vi "Autonomous Independent.vi"() -> ()   [LabVIEW 2017]
doc: "This VI is called when autonomous begins, and will automatically be terminated when autonomous ends. You can carry out timed or sensor driven robot movement independently without needing to return to the caller."
uses:
  <vilib>/Rock Robotics/WPI/Utilities/WPI_GetSetVariantRefNum.vi
  <vilib>/Rock Robotics/Network Tables/NT Read String.vi
  <vilib>/Rock Robotics/WPI/RobotDrive/WPI_RobotDriveArcadeDrive_Standard(NoSaturation).vi
  <vilib>/Rock Robotics/Network Tables/NT Write Numeric Array.vi
  Robot Global Data.vi
panel:
  out "Current Movement, for debugging":T1 {"Y Joystick Value" scale=1.0..-1.0; "X Joystick Value" scale=-1.0..1.0}
  in  "Array of robot movements":T2(array[cluster])=[{"X Joystick Value"=0.39393939393939403, "Y Joystick Value"=0.0, "Delay (sec)"=1.0, "Movement Name"="turn"}, {"X Joystick Value"=-0.3737373737373737, "Y Joystick Value"=0.0, "Delay (sec)"=1.0, "Movement Name"="turn back"}] {"Y Joystick Value" scale=1.0..-1.0; "X Joystick Value" scale=-1.0..1.0}
  # "Be sure to right-click and choose Data Operations>>Make Current Value default if you want to save the array values with the VI"
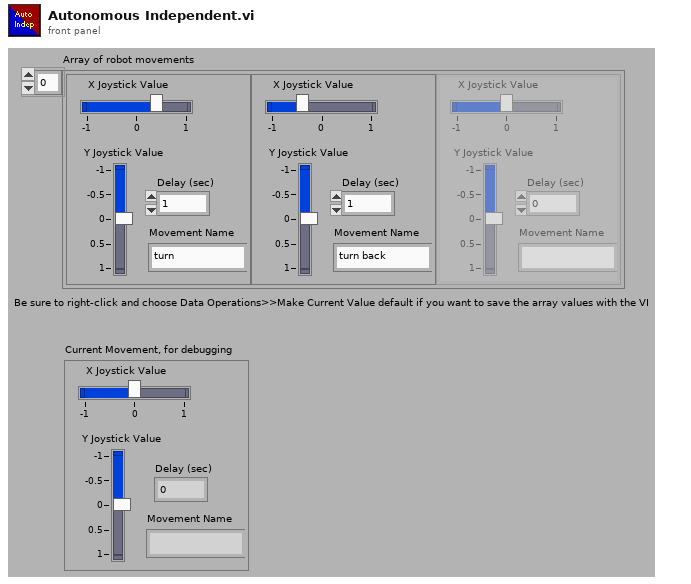
[diagram p1: front panel]
types:
  T1 = cluster{"X Joystick Value":dbl, "Y Joystick Value":dbl, "Delay (sec)":dbl, "Movement Name":string}
  T2 = cluster{"X Joystick Value":dbl, "Y Joystick Value":dbl, "Delay (sec)":dbl, "Movement Name":string}[]
  T3 = typedef "WPI_JoystickDevRef.ctl" = cluster{"Device":T4}
  T4 = typedef "WPI_JoystickDeviceEnum.ctl" = enum16{"USB 0", "USB 1", "USB 2", "USB 3", "USB 4", "USB 5"}
  T5 = typedef "WPI_RobotDriveDevRef.ctl" = cluster{"DevStatus":errorcluster, "Motors[]":T6[], "Square Inputs":bool, "Max Output":dbl}
  T6 = typedef "WPI_MotorControlDeviceRef.ctl" = cluster{"DeviceStatus":errorcluster, "Type":T7, "PWM":cluster{"PWM Channel":T8, "DeadBand":T9}, "CAN":cluster{"Device Number":u8, "SetOutput VI Ref":variant, "GetOutput VI Ref":variant, "Enable VI Ref":variant, "Disable VI Ref":variant, "Data":variant}, "Invert":bool, "DIO PWM":cluster{"PWM \"Enable\" Channel":T8, "DIOChannel":T10, "PWM Rate":dbl}}
  T7 = typedef "WPI_MotorControlType.ctl" = enum16{"PWM", "CAN", "DIO PWM"}
  T8 = typedef "FPGA_DIOPWMChannel.ctl" = enum8{"PWM 0", "PWM 1", "PWM 2", "PWM 3", "PWM 4", "PWM 5", "PWM 6", "PWM 7", "PWM 8", "PWM 9", "PWM MXP 0", "PWM MXP 1", "PWM MXP 2", "PWM MXP 3", "PWM MXP 4", "PWM MXP 5", "PWM MXP 6", "PWM MXP 7", "PWM MXP 8", "PWM MXP 9", "Invalid"}
  T9 = typedef "WPI_PWMDeadband.ctl" = cluster{"Name":string, "maxPositivePwm":i32, "minPositivePwm":i32, "centerPwm":i32, "maxNegativePwm":i32, "minNegativePwm":i32, "angularRange":u16}
  T10 = typedef "FPGA_DIOChannel.ctl" = enum8{"DIO 0", "DIO 1", "DIO 2", "DIO 3", "DIO 4", "DIO 5", "DIO 6", "DIO 7", "DIO 8", "DIO 9", "DIO MXP 0", "DIO MXP 1", "DIO MXP 2", "DIO MXP 3", "DIO MXP 4", "DIO MXP 5", "DIO MXP 6", "DIO MXP 7", "DIO MXP 8", "DIO MXP 9", "DIO MXP 10", "DIO MXP 11", "DIO MXP 12", "DIO MXP 13", "DIO MXP 14", "DIO MXP 15", "SPI Port CS1", "SPI Port CS2", "SPI Port CS3", "SPI Port MISO", "SPI Port MOSI", "Invalid"}
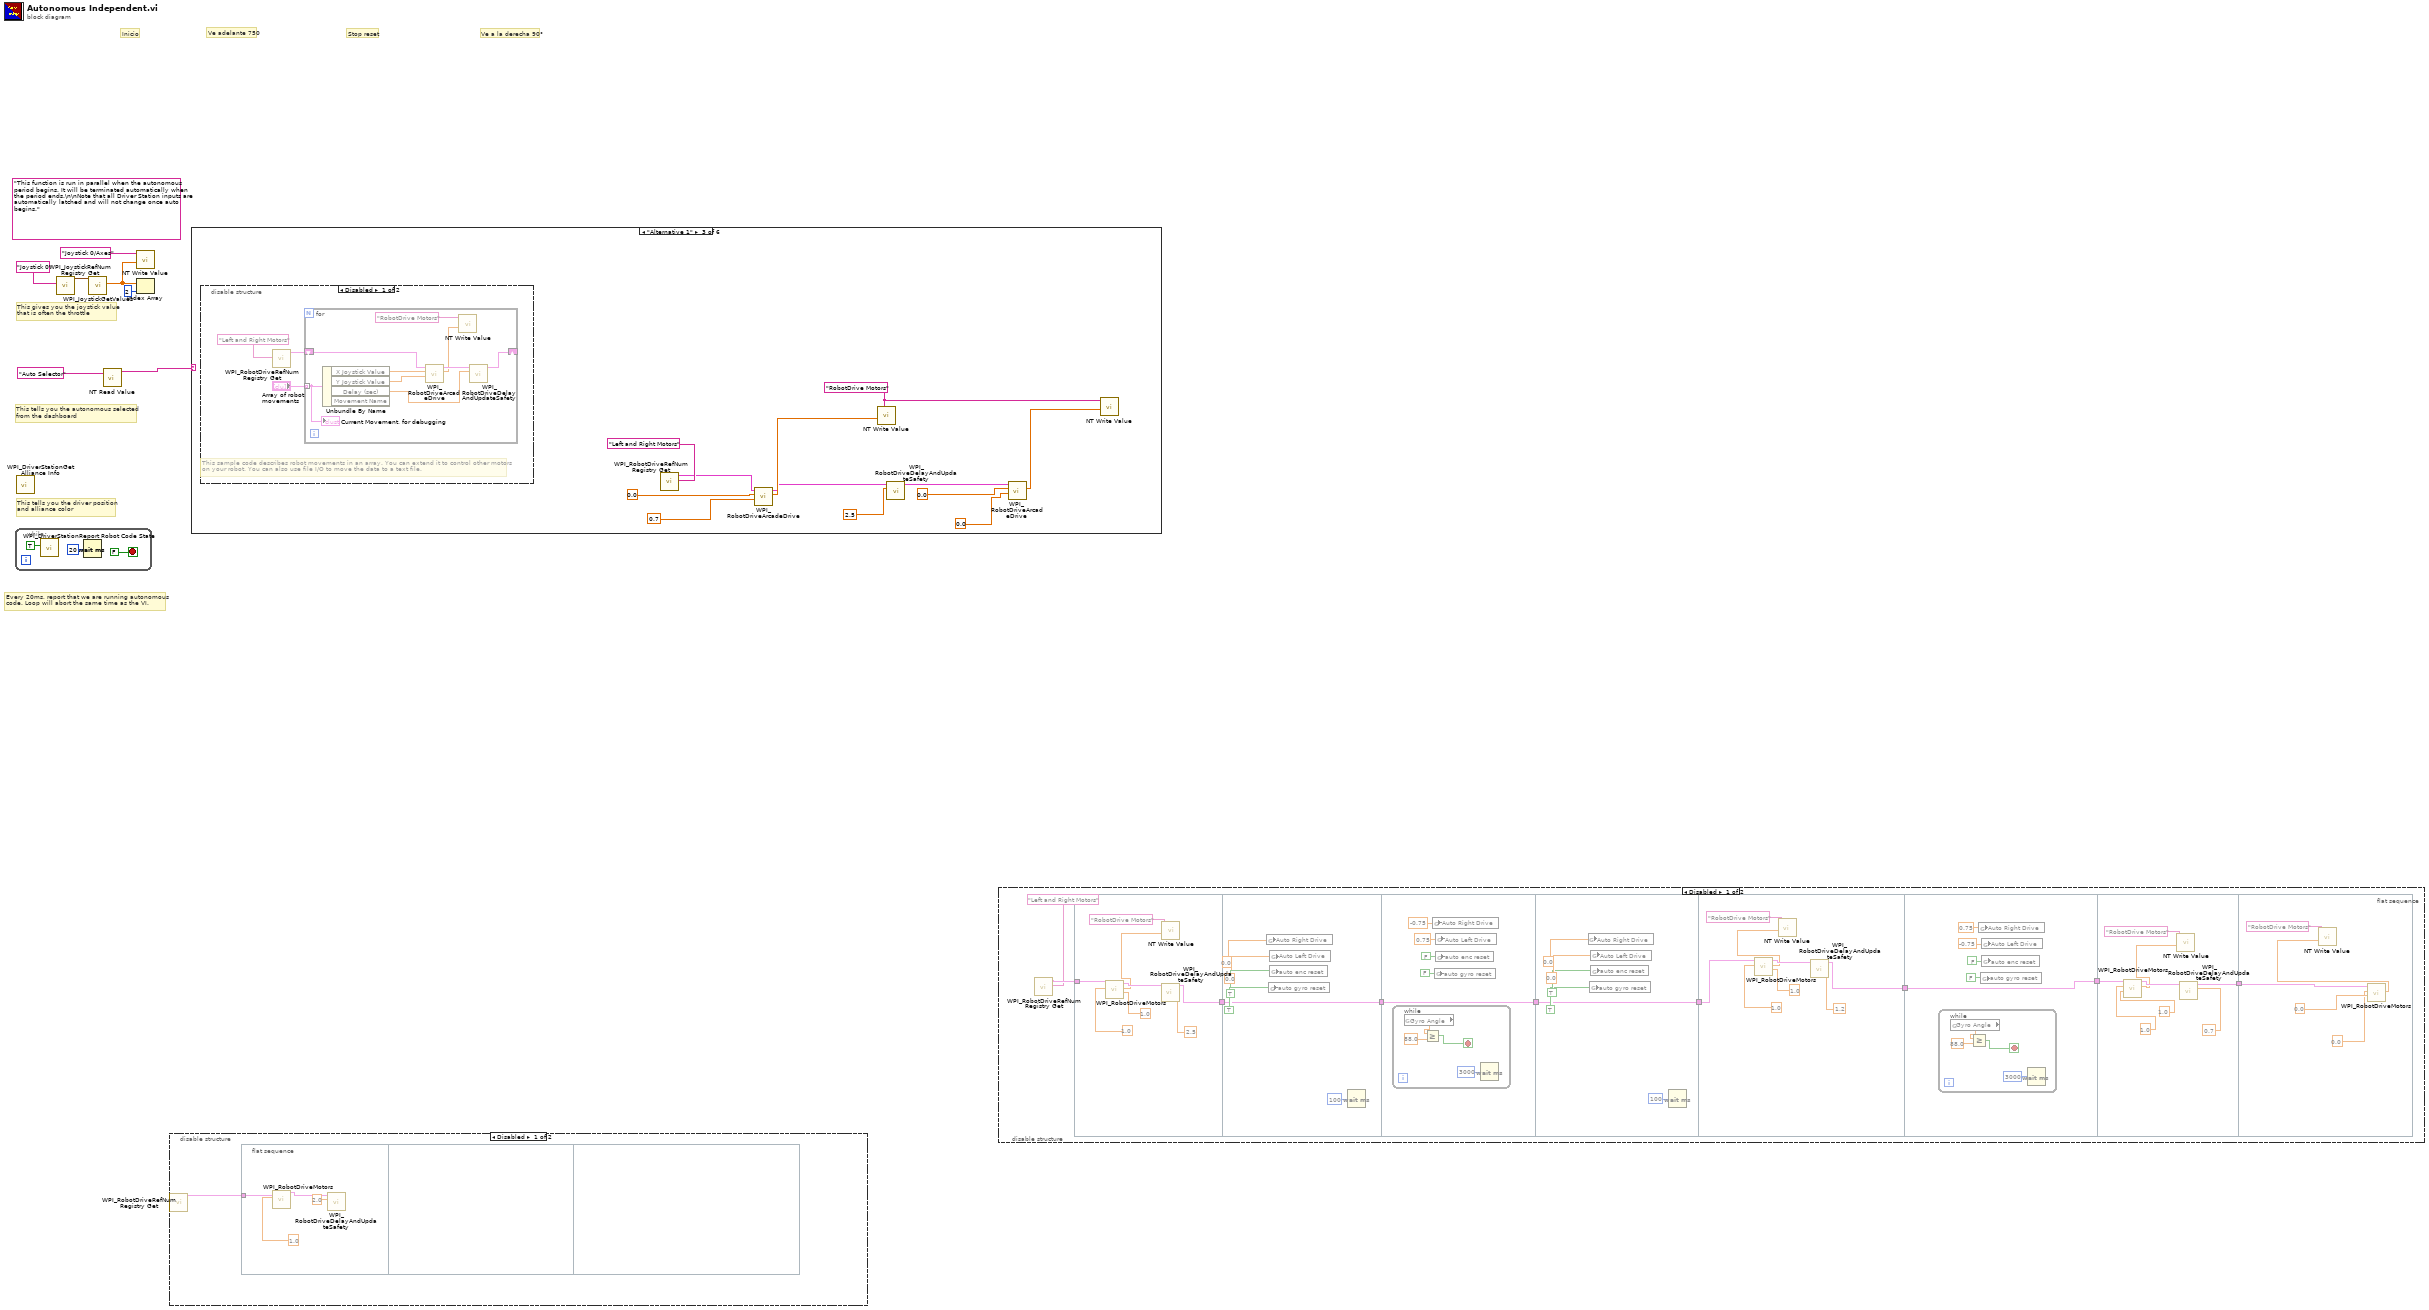
[diagram p0: block diagram]
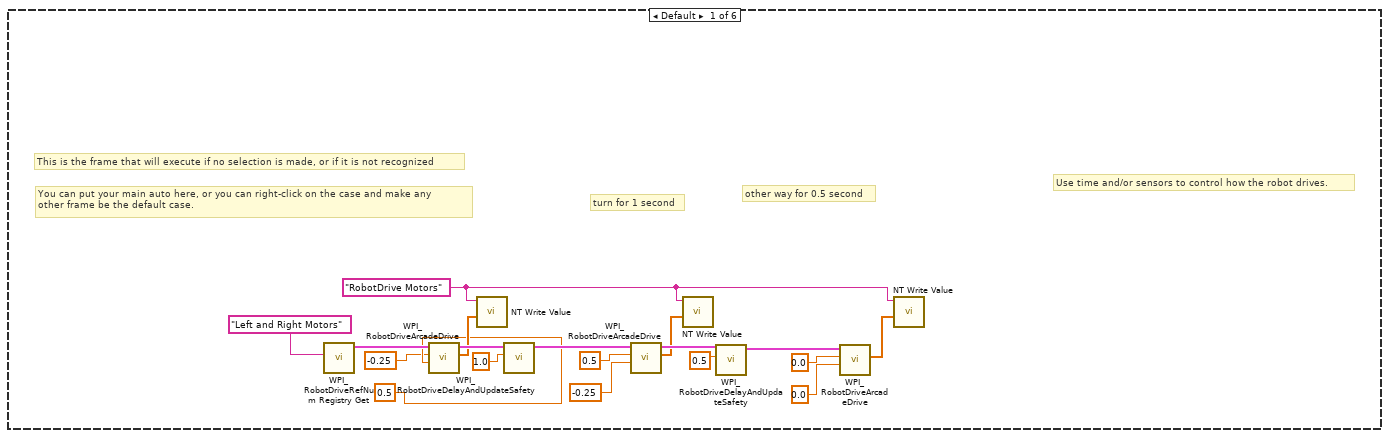
[diagram p4: hidden frame]
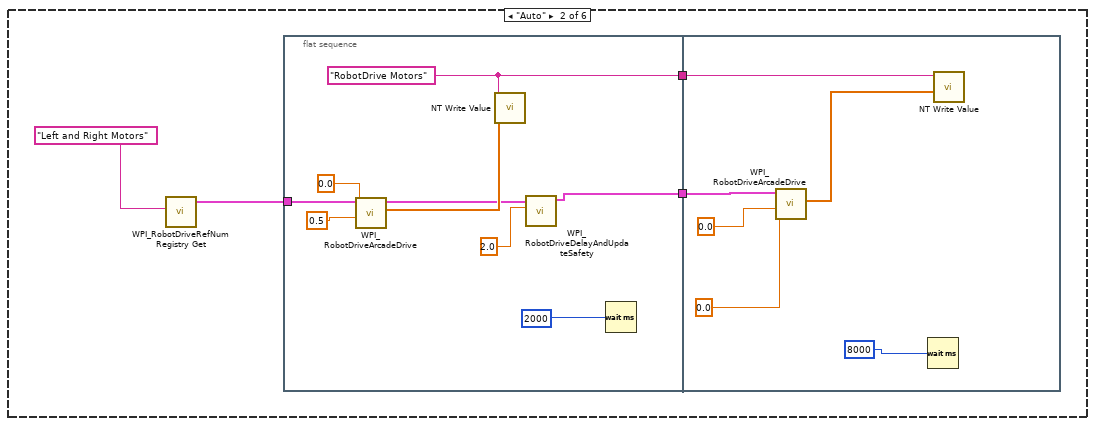
[diagram p5: hidden frame]
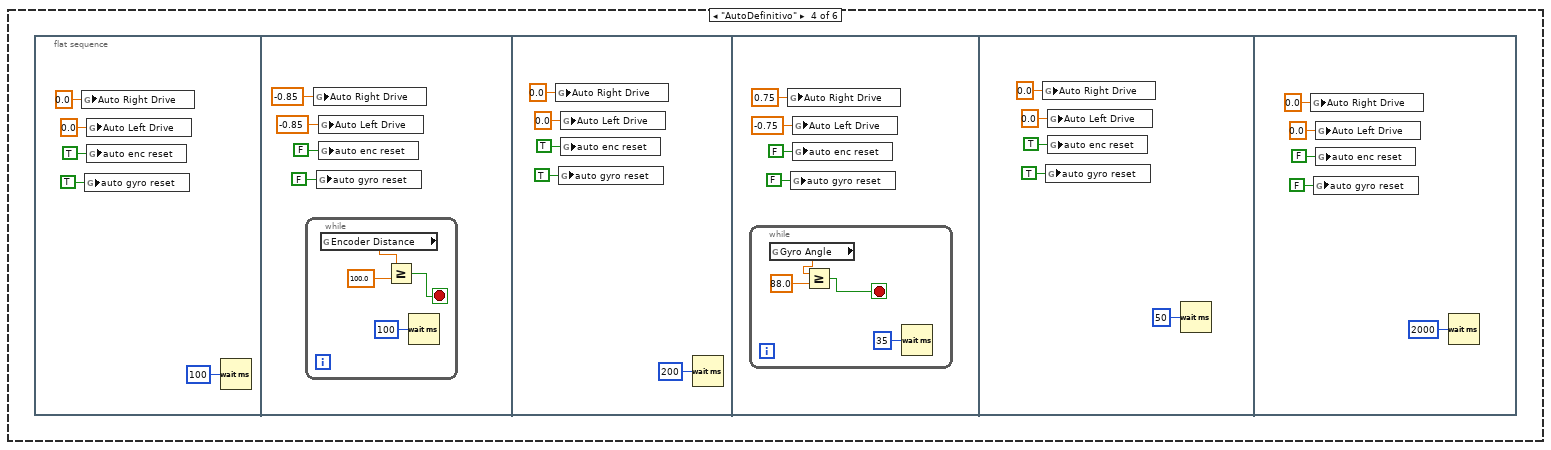
[diagram p7: hidden frame]
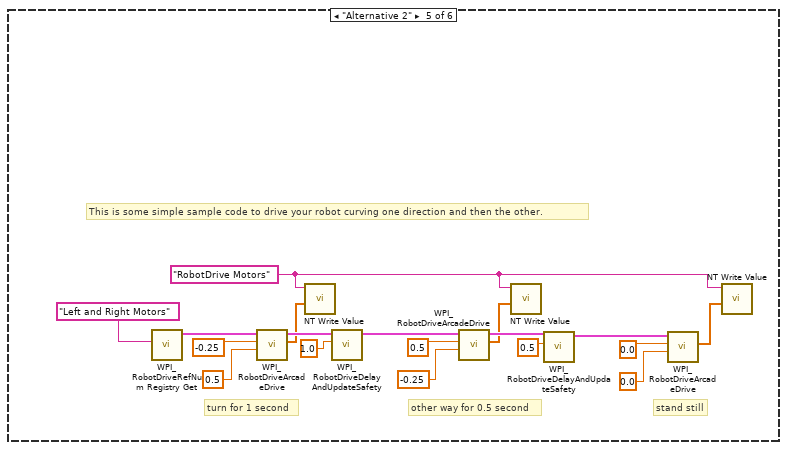
[diagram p8: hidden frame]
diagram:
  (unwired) "This function is run in parallel when the autonomous period begins. It will be terminated automatically when the period ends.\n\nNote that all Driver Station inputs are automatically latched and will not change once auto begins."
  # "Ve a la derecha 90°"
  # "Stop reset"
  # "Ve adelante 750"
  # "Inicio"
  # "This tells you the autonomous selected\nfrom the dashboard"
  # "Every 20ms, report that we are running autonomous\ncode. Loop will abort the same time as the VI."
  # "This gives you the joystick value\nthat is often the throttle"
  # "This tells you the driver position\nand alliance color"
  n1 = while {
    stop <- FALSE stop-if-true
    n2 = call <vilib>:"WPI_DriverStationReport Robot Code State.vi"("Autonomous"=TRUE) -> ()  [unwired: 10 in, 1 out]
    n3 = Wait (ms)(milliseconds to wait=u32 20) -> ()  [unwired: 1 out]
  }
  n4 = call <vilib>:"WPI_DriverStationGet Alliance Info.vi"() -> ()  [unwired: 12 out]
  n5 = call <vilib>:"WPI_JoystickRefNum Registry Get.vi"("refnum name"="Joystick 0") -> ("JoystickDevRef"=w6:T3)  [unwired: 1 in, 9 out]
  n6 = call <vilib>:"WPI_JoystickGetValues.vi"("JoystickDevRef"=w6) -> ("Axes"=w2:dbl[])  [unwired: 6 in, 4 out]
  n7 = call-poly <vilib>:"NT Read Value.vi"("Name"="Auto Selector") -> ("String"=w3:string)  [unwired: 9 in, 1 out]
  n8 = call-poly <vilib>:"NT Write Value.vi"("Numeric Array"=w2, "Name"="Joystick 0/Axes") -> ()  [unwired: 9 in, 1 out]
  n9 = Index Array(array=w2, index=2) -> ()  [unwired: 1 out]
  n10 = disable-structure shown="Disabled" {
    frame Disabled {
      n11 = call <vilib>:"WPI_RobotDriveRefNum Registry Get.vi"() -> ("RobotDriveDevRef"=w11:T5)  [unwired: 10 in, 1 out]
      n12 = flat-sequence {
        tunnel: w11 -> [w15]
        frame #0 {
          n13 = call <vilib>:"WPI_RobotDriveMotors.vi"("LeftSpeed"=1.0, "RobotDriveDevRef"=w15) -> ("RobotDriveDevRef"=w14:T5)  [unwired: 7 in, 2 out]
          n14 = call <vilib>:"WPI_RobotDriveDelayAndUpdateSafety.vi"("Delay (s)"=2.0, "RobotDriveDevRef"=w14) -> ()  [unwired: 8 in, 2 out]
        }
        frame #1 {
        }
        frame #2 {
        }
      }
    }
    frame Enabled {
    }
  }
  n15 = case shown="\"Alternative 1\"" w3 {
    frame Default {
      w25 = "RobotDrive Motors" ("Name")
      # "other way for 0.5 second"
      # "turn for 1 second"
      # "Use time and/or sensors to control how the robot drives."
      # "You can put your main auto here, or you can right-click on the case and make any\nother frame be the default case."
      # "This is the frame that will execute if no selection is made, or if it is not recognized"
      n16 = call <vilib>:"WPI_RobotDriveRefNum Registry Get.vi"("refnum name"="Left and Right Motors") -> ("RobotDriveDevRef"=w33:T5)  [unwired: 1 in, 9 out]
      n17 = call-poly <vilib>:"WPI_RobotDriveArcadeDrive.vi"("Y axis value"=0.5 ("X axis value"), "X axis value"=-0.25, "RobotDriveDevRef"=w33) -> ("Motor Values"=w26:dbl[], "RobotDriveDevRef"=w29:T5)  [unwired: 1 in, 6 out]
      n18 = call-poly <vilib>:"NT Write Value.vi"("Numeric Array"=w26, "Name"=w25) -> ()  [unwired: 9 in, 1 out]
      n19 = call <vilib>:"WPI_RobotDriveDelayAndUpdateSafety.vi"("Delay (s)"=1.0, "RobotDriveDevRef"=w29) -> ("RobotDriveDevRef 2"=w30:T5)  [unwired: 8 in, 1 out]
      n20 = call-poly <vilib>:"WPI_RobotDriveArcadeDrive.vi"("Y axis value"=-0.25 ("X axis value"), "X axis value"=0.5, "RobotDriveDevRef"=w30) -> ("Motor Values"=w27:dbl[], "RobotDriveDevRef"=w31:T5)  [unwired: 1 in, 6 out]
      n21 = call-poly <vilib>:"NT Write Value.vi"("Numeric Array"=w27, "Name"=w25) -> ()  [unwired: 9 in, 1 out]
      n22 = call <vilib>:"WPI_RobotDriveDelayAndUpdateSafety.vi"("Delay (s)"=0.5, "RobotDriveDevRef"=w31) -> ("RobotDriveDevRef 2"=w32:T5)  [unwired: 8 in, 1 out]
      n23 = call-poly <vilib>:"WPI_RobotDriveArcadeDrive.vi"("Y axis value"=0.0 ("X axis value"), "X axis value"=0.0, "RobotDriveDevRef"=w32) -> ("Motor Values"=w28:dbl[])  [unwired: 1 in, 7 out]
      n24 = call-poly <vilib>:"NT Write Value.vi"("Numeric Array"=w28, "Name"=w25) -> ()  [unwired: 9 in, 1 out]
    }
    frame "Auto" {
      n25 = call <vilib>:"WPI_RobotDriveRefNum Registry Get.vi"("refnum name"="Left and Right Motors") -> ("RobotDriveDevRef"=w36:T5)  [unwired: 9 in, 1 out]
      n26 = flat-sequence {
        tunnel: w36 -> [w46]
        tunnel: [w39] -> w35
        tunnel: [w44] -> w34
        tunnel: w35 -> [w52]
        tunnel: w34 -> [w50]
        frame #0 {
          w44 = "RobotDrive Motors" ("Name")
          n27 = call-poly <vilib>:"WPI_RobotDriveArcadeDrive.vi"("Y axis value"=0.5 ("X axis value"), "X axis value"=0.0, "RobotDriveDevRef"=w46) -> ("Motor Values"=w45:dbl[], "RobotDriveDevRef"=w41:T5)  [unwired: 6 in, 1 out]
          n28 = call-poly <vilib>:"NT Write Value.vi"("Numeric Array"=w45, "Name"=w44) -> ()  [unwired: 9 in, 1 out]
          n29 = call <vilib>:"WPI_RobotDriveDelayAndUpdateSafety.vi"("Delay (s)"=2.0, "RobotDriveDevRef"=w41) -> ("RobotDriveDevRef 2"=w39:T5)  [unwired: 8 in, 1 out]
          n30 = Wait (ms)(milliseconds to wait=2000) -> ()  [unwired: 1 out]
        }
        frame #1 {
          n31 = call-poly <vilib>:"WPI_RobotDriveArcadeDrive.vi"("Y axis value"=0.0, "X axis value"=0.0, "RobotDriveDevRef"=w52) -> ("Motor Values"=w49:dbl[])  [unwired: 6 in, 2 out]
          n32 = Wait (ms)(milliseconds to wait=8000) -> ()  [unwired: 1 out]
          n33 = call-poly <vilib>:"NT Write Value.vi"("Numeric Array"=w49, "Name"=w50) -> ()  [unwired: 9 in, 1 out]
        }
      }
    }
    frame "Alternative 1" {
      w56 = "RobotDrive Motors" ("Name")
      n34 = disable-structure shown="Disabled" {
        frame Disabled {
          # "This sample code describes robot movements in an array. You can extend it to control other motors\non your robot. You can also use file I/O to move the data to a text file."
          n35 = call <vilib>:"WPI_RobotDriveRefNum Registry Get.vi"("refnum name"="Left and Right Motors") -> ("RobotDriveDevRef"=w66:T5)  [unwired: 1 in, 9 out]
          n36 = for {
            shift-right: [w74] -> _
            shift-left: w66 -> [w75]
            tunnel: "Array of robot movements" -> [w70] mode=indexing
            n37 = Unbundle By Name(w70) -> ("X Joystick Value"=w73:dbl, "Y Joystick Value"=w72:dbl, "Delay (sec)"=w71:dbl)  [unwired: 1 out]
            n38 = call-poly <vilib>:"WPI_RobotDriveArcadeDrive.vi"("Y axis value"=w72, "X axis value"=w73, "RobotDriveDevRef"=w75) -> ("Motor Values"=w68:dbl[], "RobotDriveDevRef"=w76:T5)  [unwired: 1 in, 6 out]
            n39 = call-poly <vilib>:"NT Write Value.vi"("Numeric Array"=w68, "Name"="RobotDrive Motors") -> ()  [unwired: 9 in, 1 out]
            n40 = call <vilib>:"WPI_RobotDriveDelayAndUpdateSafety.vi"("Delay (s)"=w71, "RobotDriveDevRef"=w76) -> ("RobotDriveDevRef 2"=w74:T5)  [unwired: 8 in, 1 out]
            "Current Movement, for debugging" <- w70
          }
        }
        frame Enabled {
        }
      }
      n41 = call <vilib>:"WPI_RobotDriveRefNum Registry Get.vi"("refnum name"="Left and Right Motors") -> ("RobotDriveDevRef"=w61:T5)  [unwired: 9 in, 1 out]
      n42 = call-poly <vilib>:"WPI_RobotDriveArcadeDrive.vi"("Y axis value"=0.7 ("RightSpeed"), "X axis value"=0.0 ("LeftSpeed"), "RobotDriveDevRef"=w61) -> ("Motor Values"=w59:dbl[], "RobotDriveDevRef"=w58:T5)  [unwired: 6 in, 1 out]
      n43 = call-poly <vilib>:"NT Write Value.vi"("Numeric Array"=w59, "Name"=w56) -> ()  [unwired: 9 in, 1 out]
      n44 = call <vilib>:"WPI_RobotDriveDelayAndUpdateSafety.vi"("Delay (s)"=2.5, "RobotDriveDevRef"=w58) -> ("RobotDriveDevRef 2"=w57:T5)  [unwired: 8 in, 1 out]
      n45 = call-poly <vilib>:"WPI_RobotDriveArcadeDrive.vi"("Y axis value"=0.0 ("LeftSpeed"), "X axis value"=0.0 ("RightSpeed"), "RobotDriveDevRef"=w57) -> ("Motor Values"=w53:dbl[])  [unwired: 6 in, 2 out]
      n46 = call-poly <vilib>:"NT Write Value.vi"("Numeric Array"=w53, "Name"=w56) -> ()  [unwired: 9 in, 1 out]
    }
    frame "AutoDefinitivo" {
      n47 = flat-sequence {
        frame #0 {
          n48 = global write "Robot Global Data.vi" "Auto Right Drive"(0.0 ("Auto Right Drive")) -> ()
          n49 = global write "Robot Global Data.vi" "auto gyro reset"(TRUE ("auto gyro reset")) -> ()
          n50 = global write "Robot Global Data.vi" "Auto Left Drive"(0.0 ("Auto Left Drive")) -> ()
          n51 = global write "Robot Global Data.vi" "auto enc reset"(TRUE ("auto enc reset")) -> ()
          n52 = Wait (ms)(milliseconds to wait=u32 100) -> ()  [unwired: 1 out]
        }
        frame #1 {
          n53 = while {
            stop <- w87 stop-if-true
            n54 = global read "Robot Global Data.vi" "Encoder Distance"() -> (w89:dbl)
            n55 = Greater Or Equal?(x=w89, y=100.0) -> (x >= y?=w87:bool)
            n56 = Wait (ms)(milliseconds to wait=u32 100) -> ()  [unwired: 1 out]
          }
          n57 = global write "Robot Global Data.vi" "Auto Right Drive"(-0.85 ("Auto Right Drive")) -> ()
          n58 = global write "Robot Global Data.vi" "auto gyro reset"(FALSE ("auto gyro reset")) -> ()
          n59 = global write "Robot Global Data.vi" "Auto Left Drive"(-0.85 ("Auto Left Drive")) -> ()
          n60 = global write "Robot Global Data.vi" "auto enc reset"(FALSE ("auto enc reset")) -> ()
        }
        frame #2 {
          n61 = global write "Robot Global Data.vi" "Auto Right Drive"(0.0 ("Auto Right Drive")) -> ()
          n62 = global write "Robot Global Data.vi" "auto gyro reset"(TRUE ("auto gyro reset")) -> ()
          n63 = global write "Robot Global Data.vi" "Auto Left Drive"(0.0 ("Auto Left Drive")) -> ()
          n64 = global write "Robot Global Data.vi" "auto enc reset"(TRUE ("auto enc reset")) -> ()
          n65 = Wait (ms)(milliseconds to wait=u32 200) -> ()  [unwired: 1 out]
        }
        frame #3 {
          n66 = while {
            stop <- w100 stop-if-true
            n67 = global read "Robot Global Data.vi" "Gyro Angle"() -> (w102:dbl)
            n68 = Greater Or Equal?(x=w102, y=88.0) -> (x >= y?=w100:bool)
            n69 = Wait (ms)(milliseconds to wait=u32 35) -> ()  [unwired: 1 out]
          }
          n70 = global write "Robot Global Data.vi" "Auto Right Drive"(0.75 ("Auto Right Drive")) -> ()
          n71 = global write "Robot Global Data.vi" "auto gyro reset"(FALSE ("auto gyro reset")) -> ()
          n72 = global write "Robot Global Data.vi" "Auto Left Drive"(-0.75 ("Auto Left Drive")) -> ()
          n73 = global write "Robot Global Data.vi" "auto enc reset"(FALSE ("auto enc reset")) -> ()
        }
        frame #4 {
          n74 = global write "Robot Global Data.vi" "Auto Right Drive"(0.0 ("Auto Right Drive")) -> ()
          n75 = global write "Robot Global Data.vi" "auto gyro reset"(TRUE ("auto gyro reset")) -> ()
          n76 = global write "Robot Global Data.vi" "Auto Left Drive"(0.0 ("Auto Left Drive")) -> ()
          n77 = global write "Robot Global Data.vi" "auto enc reset"(TRUE ("auto enc reset")) -> ()
          n78 = Wait (ms)(milliseconds to wait=u32 50) -> ()  [unwired: 1 out]
        }
        frame #5 {
          n79 = global write "Robot Global Data.vi" "Auto Right Drive"(0.0 ("Auto Right Drive")) -> ()
          n80 = global write "Robot Global Data.vi" "auto gyro reset"(FALSE ("auto gyro reset")) -> ()
          n81 = global write "Robot Global Data.vi" "Auto Left Drive"(0.0 ("Auto Left Drive")) -> ()
          n82 = global write "Robot Global Data.vi" "auto enc reset"(FALSE ("auto enc reset")) -> ()
          n83 = Wait (ms)(milliseconds to wait=u32 2000) -> ()  [unwired: 1 out]
        }
      }
    }
    frame "Alternative 2" {
      w114 = "RobotDrive Motors" ("Name")
      # "This is some simple sample code to drive your robot curving one direction and then the other."
      # "stand still"
      # "other way for 0.5 second"
      # "turn for 1 second"
      n84 = call <vilib>:"WPI_RobotDriveRefNum Registry Get.vi"("refnum name"="Left and Right Motors") -> ("RobotDriveDevRef"=w130:T5)  [unwired: 1 in, 9 out]
      n85 = call-poly <vilib>:"WPI_RobotDriveArcadeDrive.vi"("Y axis value"=0.5 ("X axis value"), "X axis value"=-0.25, "RobotDriveDevRef"=w130) -> ("Motor Values"=w113:dbl[], "RobotDriveDevRef"=w123:T5)  [unwired: 1 in, 6 out]
      n86 = call-poly <vilib>:"NT Write Value.vi"("Numeric Array"=w113, "Name"=w114) -> ()  [unwired: 9 in, 1 out]
      n87 = call <vilib>:"WPI_RobotDriveDelayAndUpdateSafety.vi"("Delay (s)"=1.0, "RobotDriveDevRef"=w123) -> ("RobotDriveDevRef 2"=w124:T5)  [unwired: 8 in, 1 out]
      n88 = call-poly <vilib>:"WPI_RobotDriveArcadeDrive.vi"("Y axis value"=-0.25 ("X axis value"), "X axis value"=0.5, "RobotDriveDevRef"=w124) -> ("Motor Values"=w115:dbl[], "RobotDriveDevRef"=w125:T5)  [unwired: 1 in, 6 out]
      n89 = call-poly <vilib>:"NT Write Value.vi"("Numeric Array"=w115, "Name"=w114) -> ()  [unwired: 9 in, 1 out]
      n90 = call <vilib>:"WPI_RobotDriveDelayAndUpdateSafety.vi"("Delay (s)"=0.5, "RobotDriveDevRef"=w125) -> ("RobotDriveDevRef 2"=w126:T5)  [unwired: 8 in, 1 out]
      n91 = call-poly <vilib>:"WPI_RobotDriveArcadeDrive.vi"("Y axis value"=0.0 ("X axis value"), "X axis value"=0.0, "RobotDriveDevRef"=w126) -> ("Motor Values"=w116:dbl[])  [unwired: 1 in, 7 out]
      n92 = call-poly <vilib>:"NT Write Value.vi"("Numeric Array"=w116, "Name"=w114) -> ()  [unwired: 9 in, 1 out]
    }
    frame "Your Turn" {
    }
  }
  n93 = disable-structure shown="Disabled" {
    frame Disabled {
      n94 = call <vilib>:"WPI_RobotDriveRefNum Registry Get.vi"("refnum name"="Left and Right Motors") -> ("RobotDriveDevRef"=w132:T5)  [unwired: 9 in, 1 out]
      n95 = flat-sequence {
        tunnel: w132 -> [w144]
        tunnel: [w142] -> w139
        tunnel: w139 -> [w148]
        tunnel: [w148] -> w138
        tunnel: [w154] -> w137
        tunnel: w138 -> [w154]
        tunnel: [w163] -> w136
        tunnel: w137 -> [w163]
        tunnel: w136 -> [w172]
        tunnel: [w171] -> w135
        tunnel: [w177] -> w134
        tunnel: w135 -> [w177]
        tunnel: w134 -> [w189]
        tunnel: [w188] -> w133
        tunnel: w133 -> [w196]
        frame #0 {
          n96 = call <vilib>:"WPI_RobotDriveMotors.vi"("RightSpeed"=1.0, "LeftSpeed"=1.0, "RobotDriveDevRef"=w144) -> ("Motor Values"=w141:dbl[], "RobotDriveDevRef"=w147:T5)  [unwired: 6 in, 1 out]
          n97 = call <vilib>:"WPI_RobotDriveDelayAndUpdateSafety.vi"("Delay (s)"=2.5, "RobotDriveDevRef"=w147) -> ("RobotDriveDevRef 2"=w142:T5)  [unwired: 8 in, 1 out]
          n98 = call-poly <vilib>:"NT Write Value.vi"("Numeric Array"=w141, "Name"="RobotDrive Motors") -> ()  [unwired: 9 in, 1 out]
        }
        frame #1 {
          n99 = global write "Robot Global Data.vi" "Auto Right Drive"(0.0 ("Auto Right Drive")) -> ()
          n100 = global write "Robot Global Data.vi" "auto gyro reset"(TRUE ("auto gyro reset")) -> ()
          n101 = global write "Robot Global Data.vi" "Auto Left Drive"(0.0 ("Auto Left Drive")) -> ()
          n102 = global write "Robot Global Data.vi" "auto enc reset"(TRUE ("auto enc reset")) -> ()
          n103 = Wait (ms)(milliseconds to wait=u32 100) -> ()  [unwired: 1 out]
        }
        frame #2 {
          n104 = while {
            stop <- w160 stop-if-true
            n105 = global read "Robot Global Data.vi" "Gyro Angle"() -> (w162:dbl)
            n106 = Greater Or Equal?(x=w162, y=88.0) -> (x >= y?=w160:bool)
            n107 = Wait (ms)(milliseconds to wait=u32 3000) -> ()  [unwired: 1 out]
          }
          n108 = global write "Robot Global Data.vi" "Auto Right Drive"(-0.75 ("Auto Right Drive")) -> ()
          n109 = global write "Robot Global Data.vi" "auto gyro reset"(FALSE ("auto gyro reset")) -> ()
          n110 = global write "Robot Global Data.vi" "Auto Left Drive"(0.75 ("Auto Left Drive")) -> ()
          n111 = global write "Robot Global Data.vi" "auto enc reset"(FALSE ("auto enc reset")) -> ()
        }
        frame #3 {
          n112 = global write "Robot Global Data.vi" "Auto Right Drive"(0.0 ("Auto Right Drive")) -> ()
          n113 = global write "Robot Global Data.vi" "auto gyro reset"(TRUE ("auto gyro reset")) -> ()
          n114 = global write "Robot Global Data.vi" "Auto Left Drive"(0.0 ("Auto Left Drive")) -> ()
          n115 = global write "Robot Global Data.vi" "auto enc reset"(TRUE ("auto enc reset")) -> ()
          n116 = Wait (ms)(milliseconds to wait=u32 100) -> ()  [unwired: 1 out]
        }
        frame #4 {
          n117 = call <vilib>:"WPI_RobotDriveMotors.vi"("RightSpeed"=1.0, "LeftSpeed"=1.0, "RobotDriveDevRef"=w172) -> ("Motor Values"=w169:dbl[], "RobotDriveDevRef"=w173:T5)  [unwired: 6 in, 1 out]
          n118 = call-poly <vilib>:"NT Write Value.vi"("Numeric Array"=w169, "Name"="RobotDrive Motors") -> ()  [unwired: 9 in, 1 out]
          n119 = call <vilib>:"WPI_RobotDriveDelayAndUpdateSafety.vi"("Delay (s)"=1.2, "RobotDriveDevRef"=w173) -> ("RobotDriveDevRef 2"=w171:T5)  [unwired: 8 in, 1 out]
        }
        frame #5 {
          n120 = while {
            stop <- w183 stop-if-true
            n121 = global read "Robot Global Data.vi" "Gyro Angle"() -> (w185:dbl)
            n122 = Greater Or Equal?(x=w185, y=88.0) -> (x >= y?=w183:bool)
            n123 = Wait (ms)(milliseconds to wait=u32 3000) -> ()  [unwired: 1 out]
          }
          n124 = global write "Robot Global Data.vi" "Auto Right Drive"(0.75 ("Auto Right Drive")) -> ()
          n125 = global write "Robot Global Data.vi" "auto gyro reset"(FALSE ("auto gyro reset")) -> ()
          n126 = global write "Robot Global Data.vi" "Auto Left Drive"(-0.75 ("Auto Left Drive")) -> ()
          n127 = global write "Robot Global Data.vi" "auto enc reset"(FALSE ("auto enc reset")) -> ()
        }
        frame #6 {
          n128 = call <vilib>:"WPI_RobotDriveMotors.vi"("RightSpeed"=1.0, "LeftSpeed"=1.0, "RobotDriveDevRef"=w189) -> ("Motor Values"=w186:dbl[], "RobotDriveDevRef"=w193:T5)  [unwired: 6 in, 1 out]
          n129 = call-poly <vilib>:"NT Write Value.vi"("Numeric Array"=w186, "Name"="RobotDrive Motors") -> ()  [unwired: 9 in, 1 out]
          n130 = call <vilib>:"WPI_RobotDriveDelayAndUpdateSafety.vi"("Delay (s)"=0.7, "RobotDriveDevRef"=w193) -> ("RobotDriveDevRef 2"=w188:T5)  [unwired: 8 in, 1 out]
        }
        frame #7 {
          n131 = call <vilib>:"WPI_RobotDriveMotors.vi"("RightSpeed"=0.0, "LeftSpeed"=0.0, "RobotDriveDevRef"=w196) -> ("Motor Values"=w194:dbl[])  [unwired: 6 in, 2 out]
          n132 = call-poly <vilib>:"NT Write Value.vi"("Numeric Array"=w194, "Name"="RobotDrive Motors") -> ()  [unwired: 9 in, 1 out]
        }
      }
    }
    frame Enabled {
    }
  }
